vi "StartDaq.vi"(0 "DevicesAndSignals":T1, 5 "DaqMeasurement":refnum<k24>, 7 "SyncTimeout":i32=2000, 9 "AcquisitionMode":i32, 11 "Error in":errorcluster) -> (4 "DevicesAndSignals":T1, 6 "DaqMeasurement":refnum<k24>, 8 "MaxTimeDelta":dbl, 15 "Error out":errorcluster)   [LabVIEW 2016]
doc: "Starts (synchronized) measurement of all signals that were added to the measurement. \n\n\nDevicesAndSignal: Devices and Signals that are used for the measurement (just passed through).\nMaxTimeDelta: Maximum difference between time stamps of the first measurement values. 0 means, that the first time stamp of each signal has the same value.\nSyncTimeout: Maximum time in ms, that is used to start a synchronized measurement. If it is not possible to start a synchronized measurement within this time, an error will be thrown. \nAcquisitionMode: Modus of the data acquisition. \nSoftwareSynchronized = 0\nHardwareSynchronized = 1\nUnsynchronized = 2\nUse SoftwareSynchronized, if first timestamp of all signals should be as close as possible to each other. Therefore the devices have to be synchronized! Use HardwareSynchrnonized, if the devices are synchronized by hardware (cable) and deliver a common first timestamp for each signal. Use Unsynchronized to start a measurement without a common first timestamp for all signals (in that case syncTimeOut is not taken into account and the function returns with 0.0)"
uses:
  C:/Users/CL/Desktop/ZcDAQprj0811/ZcDAQprj/Modules/DAQ-Device/Hardware Drivers/QX/HBM LabVIEW Driver/DLLs/Hbm.Api.Common.dll
  DLLs/Hbm.Api.Common.dll
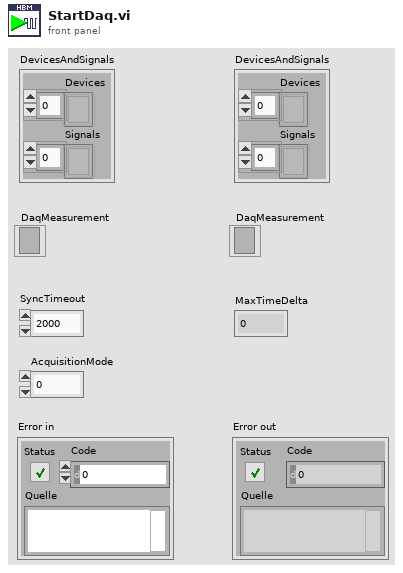
[diagram p1: front panel]
types:
  T1 = cluster{"Devices":refnum<k24>[], "Signals":refnum<k24>[]}
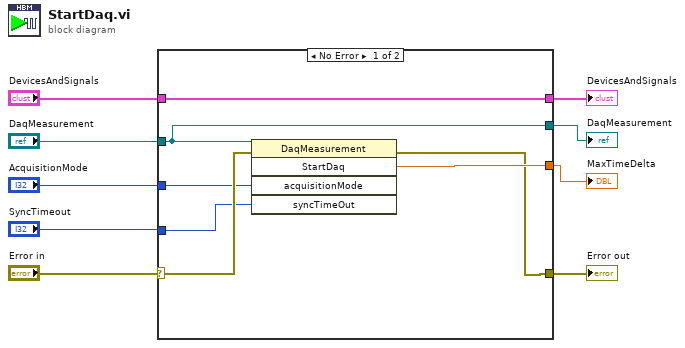
[diagram p0: block diagram]
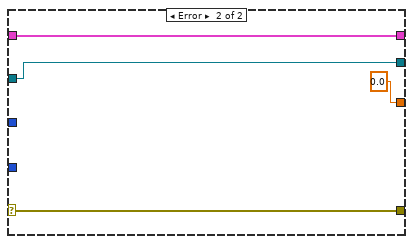
[diagram p2: hidden frame]
diagram:
  n1 = case shown="No Error" "Error in" {
    selector: "Error in" -> [w16 w20]
    tunnel: "DaqMeasurement" -> [w10 w17]
    tunnel: "DevicesAndSignals" -> [w11 w18]
    tunnel: [w12 w20] -> w6
    tunnel: "SyncTimeout" -> [w15 _]
    tunnel: "AcquisitionMode" -> [w14 _]
    tunnel: [w13 0.0 ("StartDaq")] -> w2
    tunnel: [w11 w18] -> w3
    tunnel: [w10 w17] -> w1
    frame No Error {
      n2 = invoke on="Methodenknoten" class="DaqMeasurement" method="StartDaq"(reference=w10, error in=w16, "acquisitionMode"=w14, "syncTimeOut"=w15) -> (error out=w12:errorcluster, "StartDaq"=w13:dbl)  [unwired: 1 in, 3 out]
    }
    frame Error {
    }
  }
  "Error out" <- w6
  "DevicesAndSignals" <- w3
  "MaxTimeDelta" <- w2
  "DaqMeasurement" <- w1
